vi "Sanitize Device and Axis String.vi"(11 "Device and Axis":string) -> (2 "Axis Address":string, 3 "Device Address":string)   [LabVIEW 2020, in "Zaber A Series.lvlib"]
doc: "Parses the <B>Device and Axis</B> input string and returns the Device ID and Axis ID values defined in the string. If no Device ID or Axis ID is defined in the input string then <B>0</B> is returned by default.\n\n<B>Note</B>\nThis VI does not check if the Device or Axis ID values in the input string are valid. It simply provides default values if they are not defined in the input string"
uses:
  Zaber A Series.lvlib
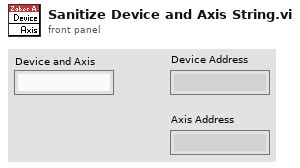
[diagram p1: front panel]
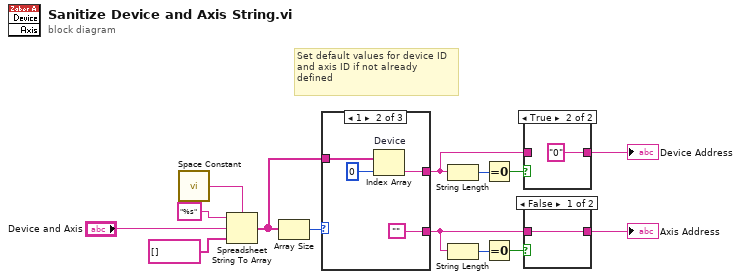
[diagram p0: block diagram]
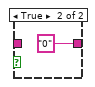
[diagram p2: hidden frame]
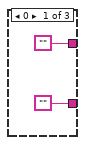
[diagram p4: hidden frame]
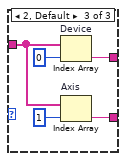
[diagram p5: hidden frame]
diagram:
  # "Set default values for device ID and axis ID if not already\ndefined"
  n1 = call <vilib>:"Space Constant.vi"() -> ("String"=w14:string)
  n2 = Spreadsheet String To Array(delimiter (Tab)=w14, format string="%s", spreadsheet string="Device and Axis", array type (2D Dbl)=string[] []) -> (array=w10:string[])
  n3 = Array Size(array=w10) -> (size(s)=w11:i32)
  n4 = case shown="1" w11 {
    tunnel: w10 -> [_ w19 w23]
    tunnel: ["" w17 w22] -> w5
    tunnel: ["" "" w21] -> w2
    frame 0 {
    }
    frame 1 {
      n5 = Index Array "Device"(array=w19, index=0) -> (element=w17:string)
    }
    frame 2, Default {
      n6 = Index Array "Device"(array=w23, index=0) -> (element=w22:string)
      n7 = Index Array "Axis"(array=w23, index=1) -> (element=w21:string)
    }
  }
  n8 = String Length(string=w5) -> (length=w8:i32)
  n9 = String Length(string=w2) -> (length=w3:i32)
  n10 = Equal To 0?(x=w8) -> (x = 0?=w7:bool)
  n11 = Equal To 0?(x=w3) -> (x = 0?=w4:bool)
  n12 = case shown="True" w7 {
    tunnel: [w26 "0"] -> w6
    tunnel: w5 -> [w26 _]
    frame False {
    }
    frame True {
    }
  }
  "Device Address" <- w6
  n13 = case shown="False" w4 {
    tunnel: [w28 "0"] -> w1
    tunnel: w2 -> [w28 _]
    frame False {
    }
    frame True {
    }
  }
  "Axis Address" <- w1
